vi "setValue.vi"(8 "error in (no error)":errorcluster, 9 "Value":variant, 10 "Key":string, 11 "Bucket in":refnum<class "Bucket.lvclass">) -> (0 "error out":errorcluster, 3 "Bucket out":refnum<class "Bucket.lvclass">)   [LabVIEW 2017, in "Bucket.lvclass"]
uses:
  <userlib>/836-Library/Data_Structures/HashMap/Support/Bucket/Bucket.lvclass
  <userlib>/836-Library/Data_Structures/HashMap/Support/Bucket/Bucket.lvclass/Bucket.ctl
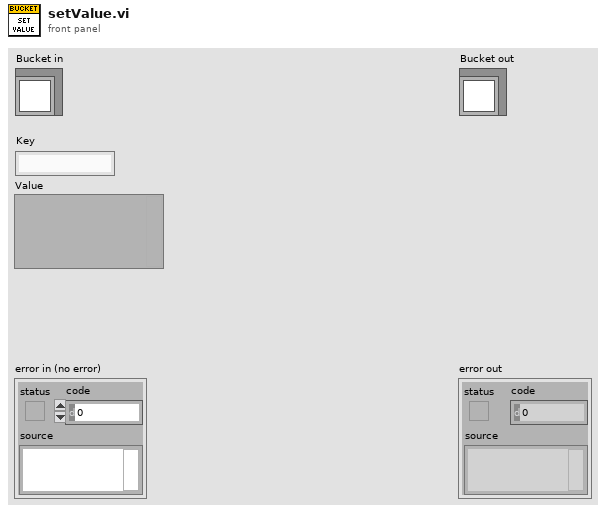
[diagram p1: front panel]
types:
  T1 = typedef "KeyValuePair.ctl" = cluster{"Key":string, "Value":variant}
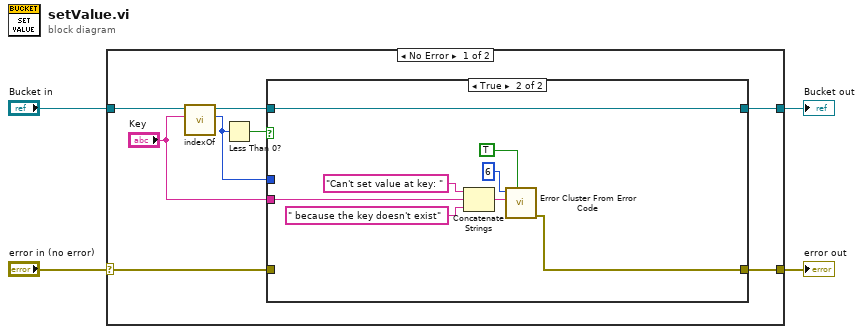
[diagram p0: block diagram]
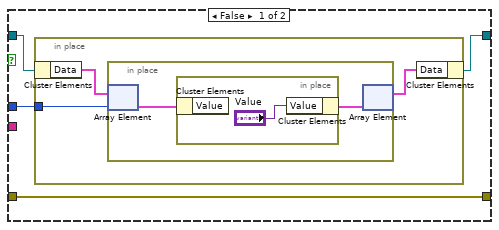
[diagram p2: hidden frame]
diagram:
  n1 = case shown="No Error" "error in (no error)" {
    selector: "error in (no error)" -> [w6 w32]
    tunnel: [w5 w32] -> w3
    tunnel: [w8 w31] -> w1
    tunnel: "Bucket in" -> [w12 w31]
    frame No Error {
      n2 = call <userlib>:"indexOf.vi"("Key"="Key", "Bucket in"=w12) -> ("Index"=w9:i32, "Bucket out"=w10:refnum<class "Bucket.lvclass">)  [unwired: 7 in, 1 out]
      n3 = Less Than 0?(x=w9) -> (x < 0?=w11:bool)
      n4 = case shown="True" w11 {
        tunnel: w10 -> [w16 w24]
        tunnel: w9 -> [w15 _]
        tunnel: [w14 w24] -> w8
        tunnel: "Key" -> [_ w27]
        tunnel: w6 -> [w13 _]
        tunnel: [w13 w23] -> w5
        frame False {
          n5 = in-place {
            in-place-border: w15 -> [w18]
            n6 = in-place-cluster #1(w16) -> ("Data"=w19:T1[])
            n7 = in-place {
              n8 = in-place-array #2(w19, w18) -> (w21:T1)
              n9 = in-place {
                n10 = in-place-cluster #3(w21) -> ()  [unwired: 1 out]
                n11 = in-place-cluster #3("Value"="Value") -> (w20:T1)
              }
              n12 = in-place-array #2(w20) -> (w17:T1[])  [unwired: 1 out]
            }
            n13 = in-place-cluster #1("Data"=w17) -> (w14:refnum<class "Bucket.lvclass">)
          }
        }
        frame True {
          n14 = Concatenate Strings("Can't set value at key: " ("string"), w27, " because the key doesn't exist" ("string")) -> (w28:string)
          n15 = call <vilib>:"Error Cluster From Error Code.vi"("show call chain? (False)"=TRUE, "error message (\"\")"=w28, "error code (0)"=6) -> ("error out"=w23:errorcluster)  [unwired: 6 in]
        }
      }
    }
    frame Error {
    }
  }
  "error out" <- w3
  "Bucket out" <- w1
